vi "Encrypt.vi"(10 "String":string, 11 "SHA-1 in":refnum<class "SHA-1.lvclass">) -> (2 "Encrypted String":string)   [LabVIEW 2020, in "User Configuration Manager.lvlib" / "SHA-1.lvclass"]
uses:
  <vilib>/gpm_packages/@cs/user-manager/Source/SHA-1 Encryption/SHA-1.lvclass
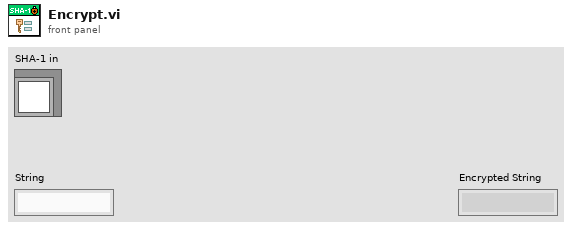
[diagram p1: front panel]
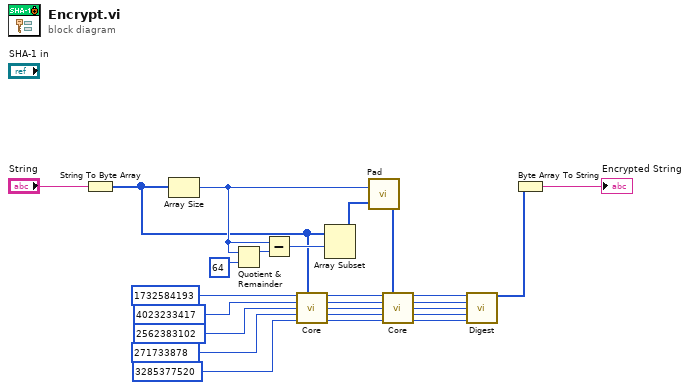
[diagram p0: block diagram]
diagram:
  n1 = String To Byte Array(string="String") -> (unsigned byte array=w3:u8[])
  n2 = Array Size(array=w3) -> (size(s)=w17:i32)
  n3 = Quotient & Remainder(x=w17, y=64) -> (x-y*floor(x/y)=w24:i32)  [unwired: 1 out]
  n4 = Subtract(x=w17, y=w24) -> (x-y=w25:i32)
  n5 = call <vilib>:"Core.vi"("s1"=u32 1732584193, "Input Bytes"=w3, "s2"=u32 4023233417, "s3"=u32 2562383102, "s4"=u32 271733878, "s5"=u32 3285377520 ("s4")) -> ("s1 out"=w14:u32, "s2 out"=w13:u32, "s3 out"=w12:u32, "s4 out"=w11:u32, "s5 out"=w10:u32)  [unwired: 5 in]
  n6 = Array Subset(array=w3, index=w25) -> (w16:u8[])  [unwired: 1 in]
  n7 = call <vilib>:"Pad.vi"("Last Part"=w16, "Message Length (bytes)"=w17) -> ("Padding"=w15:u8[])
  n8 = call <vilib>:"Core.vi"("s1"=w14, "Input Bytes"=w15, "s2"=w13, "s3"=w12, "s4"=w11, "s5"=w10) -> ("s1 out"=w9:u32, "s2 out"=w8:u32, "s3 out"=w7:u32, "s4 out"=w6:u32, "s5 out"=w5:u32)  [unwired: 5 in]
  n9 = call <vilib>:"Digest.vi"("s1"=w9, "s2"=w8, "s3"=w7, "s4"=w6, "s5"=w5) -> ("message-digest"=w2:u8[])  [unwired: 10 in]
  n10 = Byte Array To String(unsigned byte array=w2) -> (string=→"Encrypted String":string)
